vi "Abort.vi"   [LabVIEW 2017]
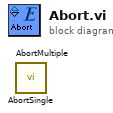
[diagram p0: block diagram]
diagram:
  n1 = call "AbortMultiple.vi"() -> ()  [unwired: 10 in, 2 out]
  n2 = call "AbortSingle.vi"() -> ()  [unwired: 10 in, 2 out]
